vi "Configure Module.vi"(8 "error in (no error)":errorcluster, 11 "Rename in":refnum<class "Rename.lvclass">) -> (0 "error out":errorcluster, 2 "Changed":bool, 3 "Rename out":refnum<class "Rename.lvclass">)   [LabVIEW 2015, in "Generic Module Library.lvlib" / "Template G_Module.lvlib" / "Rename.lvclass"]
uses:
  Rename.lvclass
  Private API/Module Control Manager/Control_Mgr_Class/Controls_Mgr.lvclass
panel:
  in  "Config XML":string
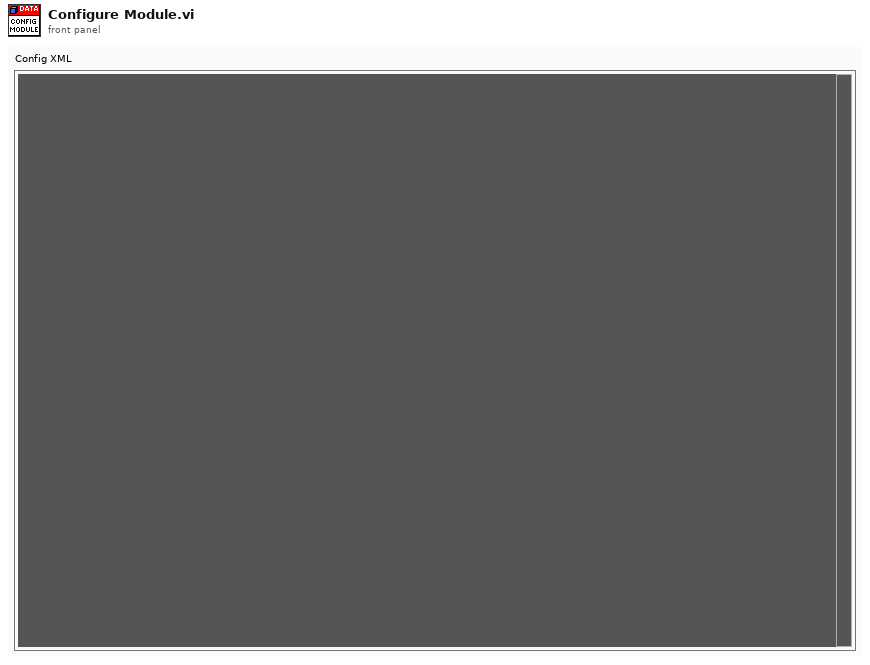
[diagram p1: front panel]
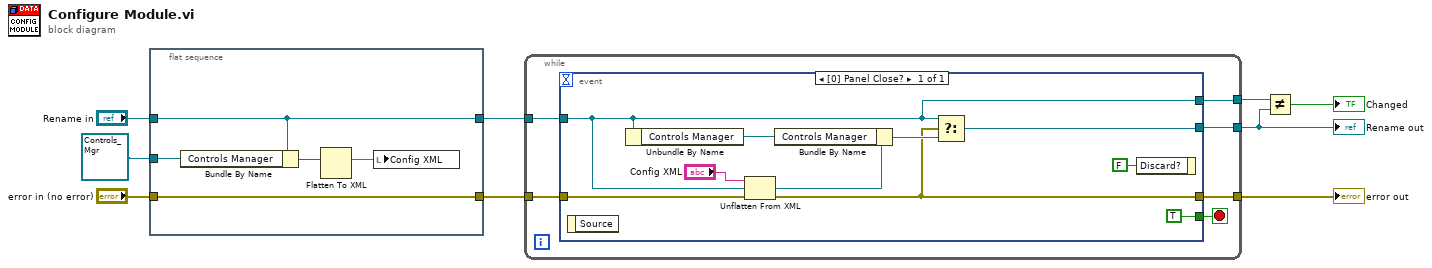
[diagram p0: block diagram]
diagram:
  n1 = flat-sequence {
    tunnel: "Rename in" -> [w10]
    tunnel: [w10] -> w6
    tunnel: "error in (no error)" -> [w14]
    tunnel: [w14] -> w7
    tunnel: refnum<class "Controls_Mgr.lvclass"> refnum ("Controls Manager") -> [w11]
    frame #0 {
      n2 = Bundle By Name(cluster=w10, "Controls Manager"=w11) -> (w12:refnum<class "Rename.lvclass">)
      n3 = Flatten To XML(anything=w12) -> (xml string=w13:string)
      n4 = local write "Config XML"(w13) -> ()
    }
  }
  n5 = while {
    tunnel: w7 -> [w20]
    tunnel: w6 -> [w18]
    tunnel: [w16] -> w3
    tunnel: [w17] -> w4
    tunnel: [w15] -> w2
    stop <- w19 stop-if-true
    n6 = event shown="[0] Panel Close?" {
      selector: _ -> [_]
      dyn-events: _ -> [_]
      timeout: _ -> [_]
      tunnel: w20 -> [w28]
      tunnel: [TRUE] -> w19
      tunnel: w18 -> [w21]
      tunnel: [w26] -> w16
      tunnel: [w23] -> w17
      tunnel: [w21] -> w15
      event Panel Close? {
        n7 = event-data() -> ()  [unwired: 1 in, 1 out]
        n8 = Unbundle By Name(w21) -> ("Controls Manager"=w24:refnum<class "Controls_Mgr.lvclass">)
        n9 = Unflatten From XML(xml string="Config XML", type=w21, error in (no error)=w28) -> (value=w27:refnum<class "Rename.lvclass">, error out=w23:errorcluster)
        n10 = Bundle By Name(cluster=w27, "Controls Manager"=w24) -> (w25:refnum<class "Rename.lvclass">)
        n11 = Select(t=w21, s=w23, f=w25) -> (s? t:f=w26:refnum<class "Rename.lvclass">)
        n12 = event-data("Discard?"=FALSE) -> ()  [unwired: 1 in, 1 out]
      }
    }
  }
  "error out" <- w4
  "Rename out" <- w3
  n13 = Not Equal?(x=w2, y=w3) -> (x != y?=→"Changed":bool)
